vi "calibrate_ref.vi"(6 "Reset":bool, 8 "Config":T2={"IO params"={"Conversion"={"Rate"=4.0, "In cards"=2, "Out channels"=4}, "Carriers"={"Phase shift"=180.0, "Levels"=[[0.8, 0.8, 0.8], [0.03, 0.03, 0.03]], "Delay samples"=73.15}}, "High rate STFT"={"Win param"=101.5, "Window type"=61, "Win order"=2, "DFT size"=64, "Channels"=[7], "Oversample"=64}, "Low rate STFT"={"Win param"=120.0, "Window type"=61, "Win order"=8, "DFT size"=64, "Channels"=[7], "Oversample"=64}, "Filtering"={"Hum"={"Frequency"=0.0, "Tc"=0.0, "Limit"=101.5, "FFT filter"=FALSE, "Detrend mode"=enum."Robust linear", "Enable"=FALSE}, "Kalman"={"Process noise"=101.5, "Measure noise"=101.5}, "Distortion"={"LF cut"=101.5, "Tc"=3.0, "Limit"=101.5, "FFT filter"=FALSE, "Detrend mode"=enum."Robust linear", "Enable"=FALSE}}} {"Filtering"."Distortion"."Limit" format="%#_3p"; "Filtering"."Distortion"."LF cut" format="%#_3p"; "Filtering"."Kalman"."Measure noise" format="%#_3p"; "Filtering"."Kalman"."Process noise" format="%#_3p"; "Filtering"."Hum"."Limit" format="%#_3p"; "Filtering"."Hum"."Frequency" format="%#_4p"; "Low rate STFT"."Oversample" min=1 step=1; "Low rate STFT"."Channels" min=0 step=1; "Low rate STFT"."DFT size" min=1 step=1; "Low rate STFT"."Window type" items=["Rectangle"=0, "Hanning"=1, "Hamming"=2, "Blackman-Harris"=3, "Exact Blackman"=4, "Blackman"=5, "Flat Top"=6, "4 Term B-Harris "=7, "7 Term B-Harris"=8, "Low Sidelobe"=9, "Blackman Nuttall"=11, "Triangle"=30, "Bartlett-Hanning"=31, "Bohman"=32, "Parzen"=33, "Welch"=34, "Kaiser"=60, "Dolph-Chebyshev"=61, "Gaussian"=62]; "High rate STFT"."Oversample" min=1 step=1; "High rate STFT"."Channels" min=0 step=1; "High rate STFT"."DFT size" min=1 step=1; "High rate STFT"."Window type" items=["Rectangle"=0, "Hanning"=1, "Hamming"=2, "Blackman-Harris"=3, "Exact Blackman"=4, "Blackman"=5, "Flat Top"=6, "4 Term B-Harris "=7, "7 Term B-Harris"=8, "Low Sidelobe"=9, "Blackman Nuttall"=11, "Triangle"=30, "Bartlett-Hanning"=31, "Bohman"=32, "Parzen"=33, "Welch"=34, "Kaiser"=60, "Dolph-Chebyshev"=61, "Gaussian"=62]; "IO params"."Carriers"."Levels" min=0.0 step=0.1; "IO params"."Conversion"."Rate" format="%#_8g"}, 9 "Modulation info":T1={"Fs full"=0.0, "Fs high"=0.0, "Fs low"=0.0, "Read size"=5000, "FFT size low"=5000, "df low"=5000.0, "High carriers"=[], "Low carriers"=[], "Hi channels at low"=[7]} {"Hi channels at low" min=0 step=1; "Low carriers" format="%#_6p"; "High carriers" format="%#_6p"}, 11 "data in":waveform(dbl)[][](array[waveform])) -> (0 "Clipping":bool, 1 "I RMS":dbl[](array[numeric]) format="%.3g", 3 "Raw data":dbl[][][](array[numeric]))   [LabVIEW 2014]
uses:
  ilemt_config.ctl
  IO_params.ctl
  stft_params.ctl
  <vilib>/Analysis/4window.llb/windowTd.ctl
  filter_params.ctl
  detrend_mode.ctl
  modulation_info.ctl
  <vilib>/Analysis/NI_AALPro.lvlib
panel:
  in  "Full scale current (A)":dbl[](array[numeric])=[16.34, 16.34, 16.34]
  # "Page is the card number, where current sense is card 0, and later cards are for sensors.  The row is XYZ and the column is sample."
  # "Make ref channel be calibrated in amps and convert data from waveform array to 3D array."
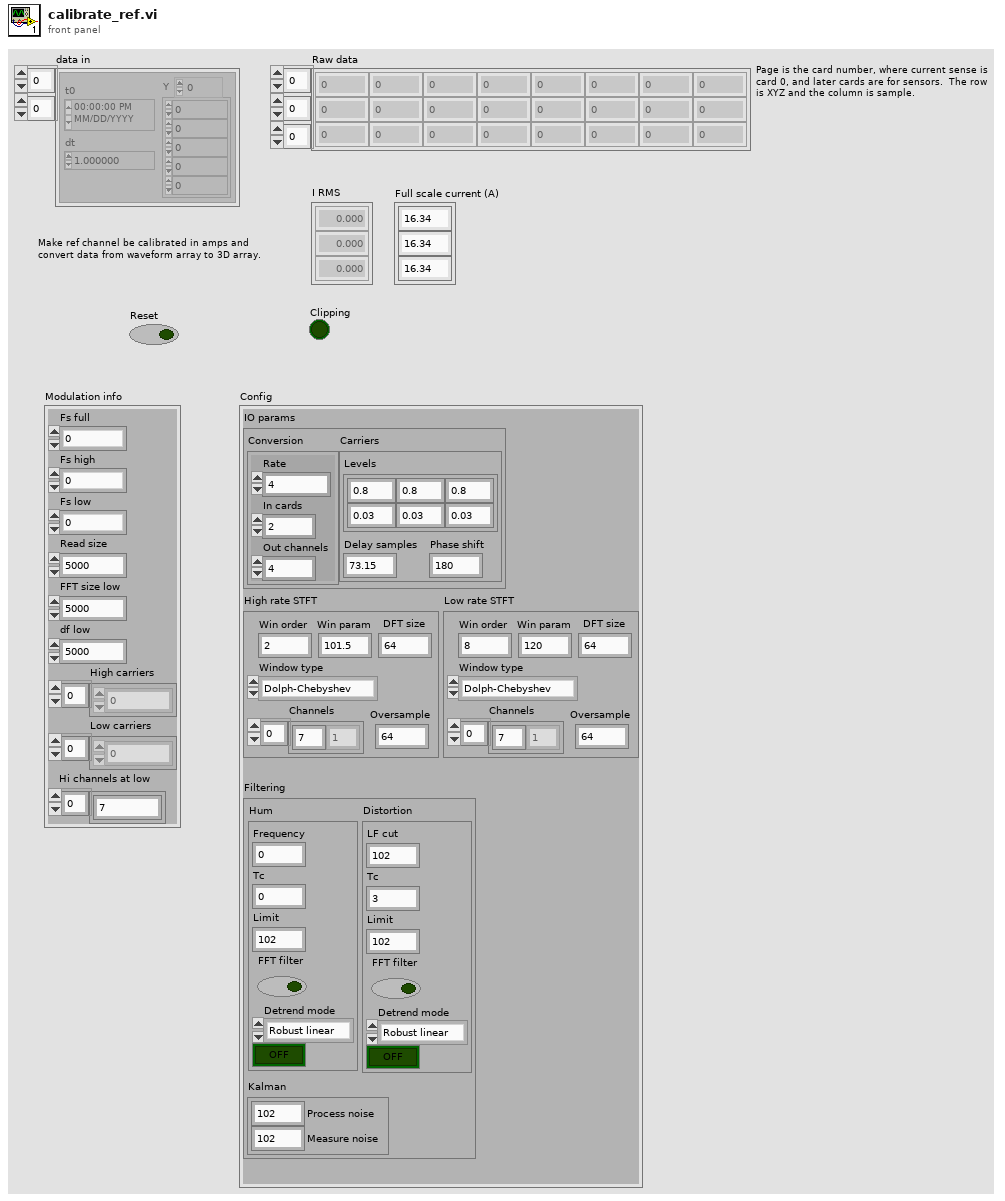
[diagram p1: front panel]
types:
  T1 = typedef "modulation_info.ctl" = cluster{"Fs full":dbl, "Fs high":dbl, "Fs low":dbl, "Read size":i32, "FFT size low":i32, "df low":dbl, "High carriers":dbl[], "Low carriers":dbl[], "Hi channels at low":i32[]}
  T2 = typedef "ilemt_config.ctl" = cluster{"IO params":T3, "High rate STFT":T4, "Low rate STFT":T4, "Filtering":T6}
  T3 = typedef "IO_params.ctl" = cluster{"Conversion":cluster{"Rate":dbl, "In cards":u32, "Out channels":u32}, "Carriers":cluster{"Phase shift":dbl, "Levels":dbl[][], "Delay samples":dbl}}
  T4 = typedef "stft_params.ctl" = cluster{"Win param":dbl, "Window type":T5, "Win order":i32, "DFT size":i32, "Channels":i32[], "Oversample":i32}
  T5 = typedef "NI_AALPro.lvlib/windowTd.ctl" = u32
  T6 = typedef "filter_params.ctl" = cluster{"Hum":cluster{"Frequency":dbl, "Tc":dbl, "Limit":dbl, "FFT filter":bool, "Detrend mode":T7, "Enable":bool}, "Kalman":cluster{"Process noise":dbl, "Measure noise":dbl}, "Distortion":cluster{"LF cut":dbl, "Tc":dbl, "Limit":dbl, "FFT filter":bool, "Detrend mode":T7, "Enable":bool}}
  T7 = typedef "detrend_mode.ctl" = enum16{"Zero mean", "Linear", "Robust linear"}
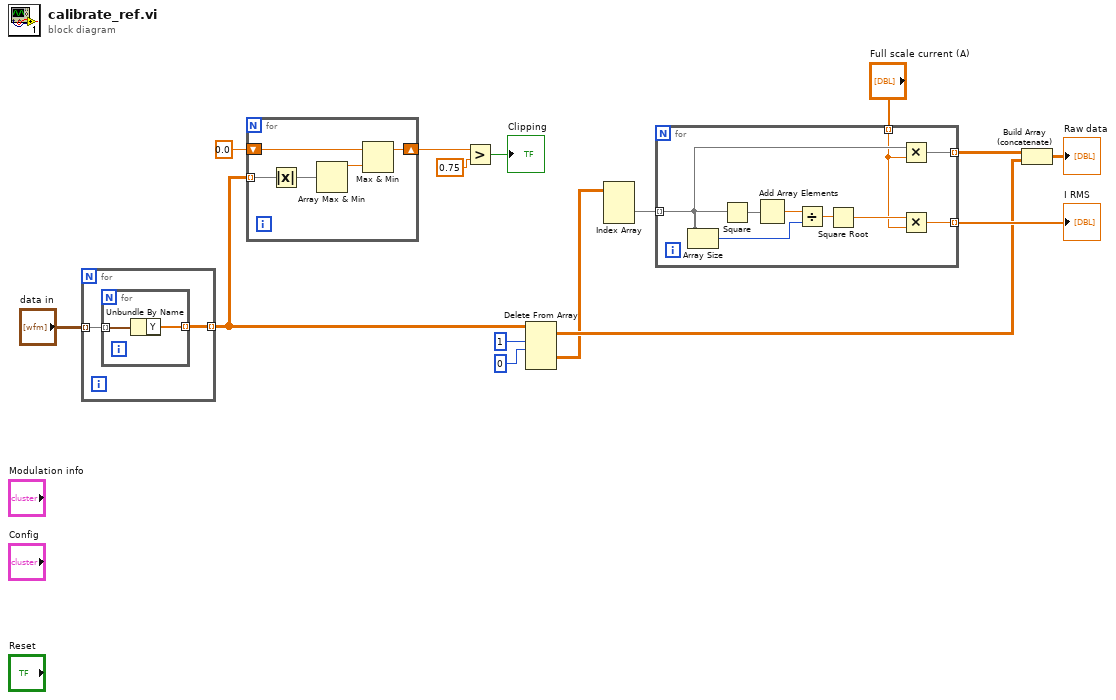
[diagram p0: block diagram]
diagram:
  n1 = for {
    tunnel: "data in" -> [w17] mode=indexing
    tunnel: [w16] -> w4 mode=indexing
    n2 = for {
      tunnel: w17 -> [w19] mode=indexing
      tunnel: [w18] -> w16 mode=indexing
      n3 = Unbundle By Name(w19) -> ("Y"=w18:dbl[])
    }
  }
  n4 = for {
    tunnel: w4 -> [w21] mode=indexing
    shift-right: [w22] -> w9
    shift-left: 0.0 -> [w23]
    n5 = Absolute Value(x=w21) -> (abs(x)=w20:dbl[][])
    n6 = Array Max & Min(array=w20) -> (max value=w24:dbl)  [unwired: 3 out]
    n7 = Max & Min(x=w23, y=w24) -> (max(x,y)=w22:dbl)  [unwired: 1 out]
  }
  n8 = Greater?(x=w9, y=0.75) -> (0:→"Clipping":bool)
  n9 = Delete From Array(array=w4, length=1, index (dim 0)=0 ("index (row)")) -> (deleted portion=w2:dbl[][][], array with subset deleted=w5:dbl[][][])  [unwired: 2 in]
  n10 = Index Array(array=w2) -> (element=w1:dbl[][])  [unwired: 3 in]
  n11 = for {
    tunnel: [w29] -> w14 mode=indexing
    tunnel: [w28] -> w6 mode=indexing
    tunnel: w1 -> [w27] mode=indexing
    tunnel: "Full scale current (A)" -> [w25] mode=indexing
    n12 = Array Size(array=w27) -> (size(s)=w33:i32)
    n13 = Square(x=w27) -> (x^2=w30:dbl[])
    n14 = Add Array Elements(numeric array=w30) -> (sum=w31:dbl)
    n15 = Divide(x=w31, y=w33) -> (x/y=w32:dbl)
    n16 = Square Root(x=w32) -> (sqrt(x)=w26:dbl)
    n17 = Multiply(x=w27, y=w25) -> (x*y=w28:dbl[])
    n18 = Multiply(x=w26, y=w25) -> (x*y=w29:dbl)
  }
  "I RMS" <- w14
  n19 = Build Array (concatenate)(w6, w5) -> (→"Raw data":dbl[][][])
